vi "粘贴.vi"(8 "error in (no error)":errorcluster caption="错误输入（无错误）", 11 "程序 输入":refnum<class "程序.lvclass">) -> (0 "error out":errorcluster caption="错误输出", 3 "程序 输出":refnum<class "程序.lvclass">)   [LabVIEW 2020, in "程序.lvclass"]
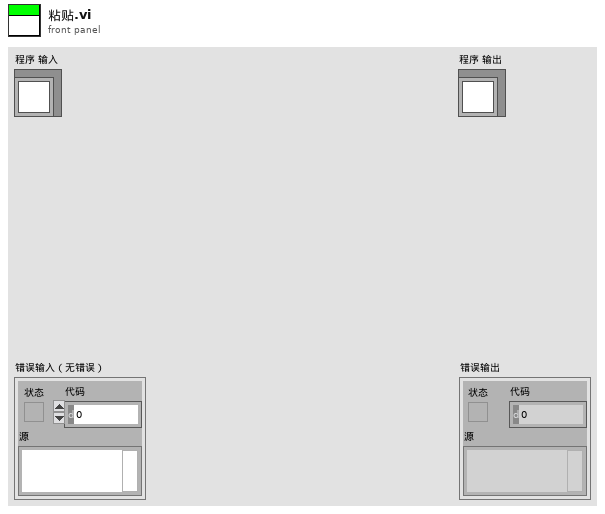
[diagram p1: front panel]
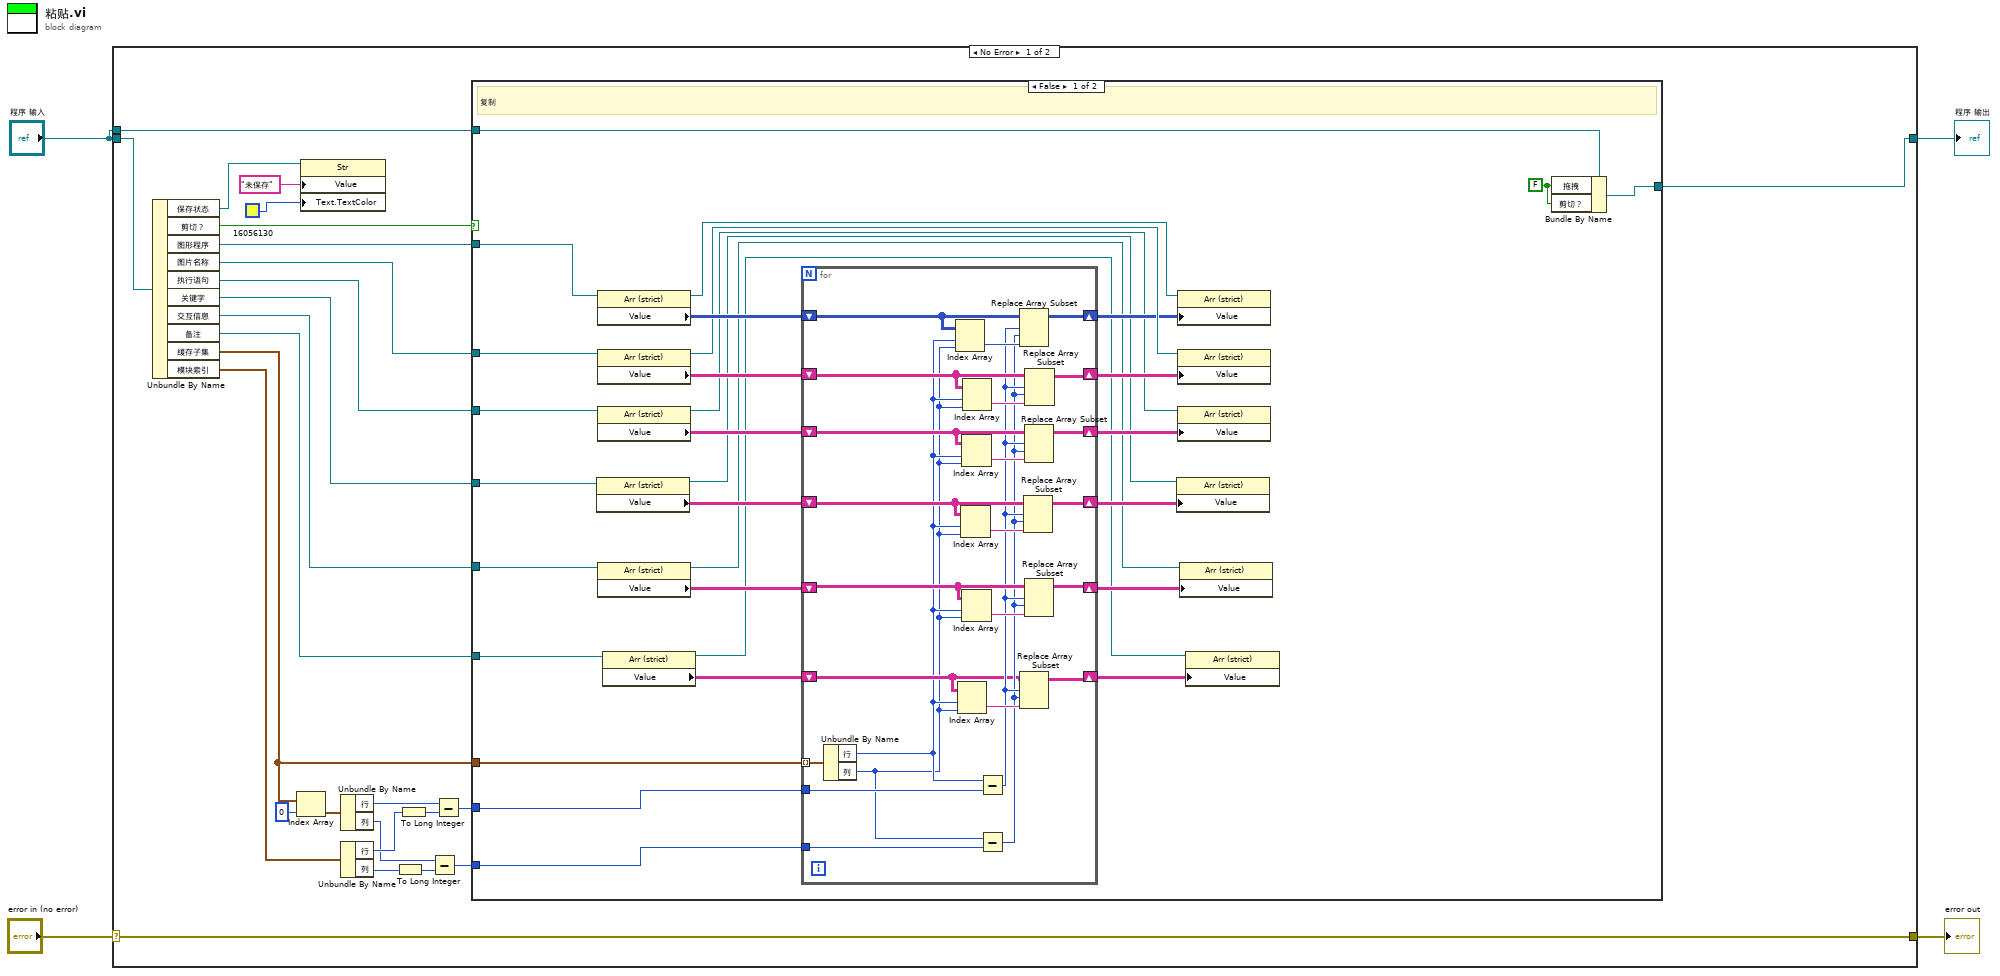
[diagram p0: block diagram]
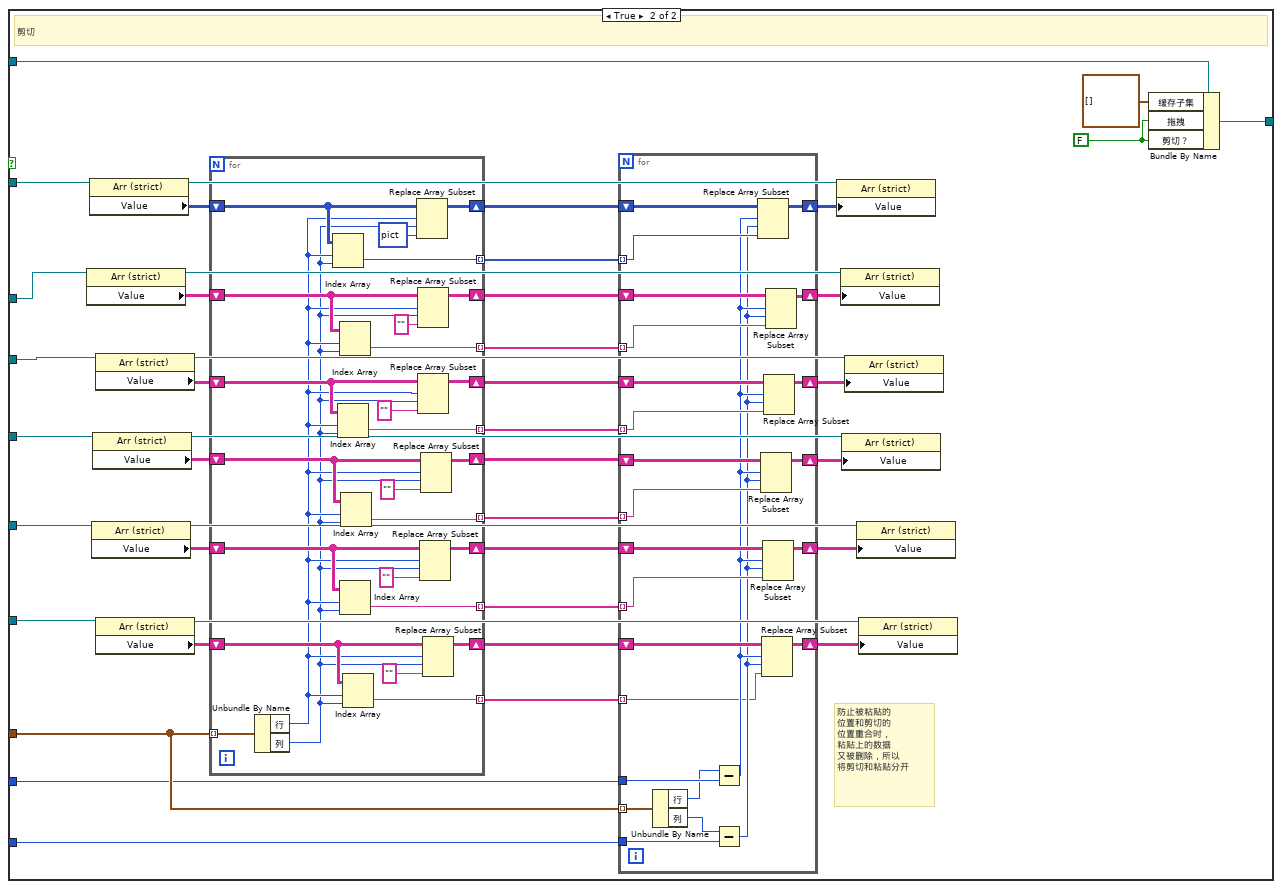
[diagram p2: hidden frame]
diagram:
  n1 = case shown="No Error" "error in (no error)" {
    selector: "error in (no error)" -> [w30 w182]
    tunnel: [w30 w182] -> w3
    tunnel: [w5 w181] -> w2
    tunnel: "程序 输入" -> [w7 w181]
    tunnel: "程序 输入" -> [w6 _]
    frame No Error {
      n2 = Unbundle By Name(w7) -> ("保存状态"=w8:refnum<vi>, "剪切？"=w19:bool, "图形程序"=w18:refnum<vi>, "图片名称"=w17:refnum<vi>, "执行语句"=w16:refnum<vi>, "关键字"=w13:refnum<vi>, "交互信息"=w12:refnum<vi>, "备注"=w11:refnum<vi>, "缓存子集"=w14:cluster{"行":i32, "列":i32}[], "模块索引"=w15:cluster{"列":u32, "行":u32})
      n3 = Index Array(array=w14, index=0 ("索引")) -> (element=w29:cluster{"行":i32, "列":i32})
      n4 = property class="Str"(reference=w8, "Value"="未保存" ("值"), "Text.TextColor"=u32 16056130) -> ()  [unwired: 1 in, 2 out]
      n5 = Unbundle By Name(w29) -> ("行"=w28:i32, "列"=w24:i32)
      n6 = Unbundle By Name(w15) -> ("行"=w27:u32, "列"=w23:u32)
      n7 = To Long Integer(number=w23) -> (32bit integer=w25:i32)
      n8 = To Long Integer(number=w27) -> (32bit integer=w26:i32)
      n9 = Subtract(x=w24, y=w25) -> (x-y=w21:i32)
      n10 = Subtract(x=w28, y=w26) -> (x-y=w22:i32)
      n11 = case shown="False" w19 {
        tunnel: w18 -> [w57 w121]
        tunnel: w17 -> [w55 w119]
        tunnel: w16 -> [w53 w116]
        tunnel: w14 -> [w58 w128]
        tunnel: w22 -> [w60 w124]
        tunnel: w21 -> [w59 w123]
        tunnel: w13 -> [w43 w106]
        tunnel: w12 -> [w41 w101]
        tunnel: w11 -> [w37 w95]
        tunnel: w6 -> [w33 w89]
        tunnel: [w32 w86] -> w5
        frame False {
          w31 = FALSE ("拖拽")
          # "复制"
          n12 = property class="Arr (strict)"(reference=w43) -> (reference out=w42:refnum<vi>, "Value"=w44:string[][])  [unwired: 1 in, 1 out]
          n13 = property class="Arr (strict)"(reference=w57) -> (reference out=w51:refnum<vi>, "Value"=w56:picture[][])  [unwired: 1 in, 1 out]
          n14 = property class="Arr (strict)"(reference=w55) -> (reference out=w48:refnum<vi>, "Value"=w54:string[][])  [unwired: 1 in, 1 out]
          n15 = property class="Arr (strict)"(reference=w53) -> (reference out=w46:refnum<vi>, "Value"=w52:string[][])  [unwired: 1 in, 1 out]
          n16 = property class="Arr (strict)"(reference=w41) -> (reference out=w39:refnum<vi>, "Value"=w40:string[][])  [unwired: 1 in, 1 out]
          n17 = property class="Arr (strict)"(reference=w37) -> (reference out=w34:refnum<vi>, "Value"=w36:string[][])  [unwired: 1 in, 1 out]
          n18 = for {
            tunnel: w58 -> [w85] mode=indexing
            tunnel: w60 -> [w84]
            tunnel: w59 -> [w83]
            shift-right: [w78] -> w47
            shift-left: w56 -> [w79]
            shift-right: [w76] -> w50
            shift-left: w54 -> [w77]
            shift-right: [w74] -> w49
            shift-left: w52 -> [w75]
            shift-right: [w73] -> w45
            shift-left: w44 -> [w72]
            shift-right: [w69] -> w38
            shift-left: w40 -> [w68]
            shift-right: [w66] -> w35
            shift-left: w36 -> [w63]
            n19 = Unbundle By Name(w85) -> ("行"=w62:i32, "列"=w61:i32)
            n20 = Index Array(array=w79, index (row)=w62, index (col)=w61) -> (element=w82:picture)
            n21 = Index Array(array=w63, index (row)=w62, index (col)=w61) -> (element=w67:string)
            n22 = Index Array(array=w72, index (row)=w62, index (col)=w61) -> (element=w71:string)
            n23 = Index Array(array=w75, index (row)=w62, index (col)=w61) -> (element=w80:string)
            n24 = Index Array(array=w68, index (row)=w62, index (col)=w61) -> (element=w70:string)
            n25 = Index Array(array=w77, index (row)=w62, index (col)=w61) -> (element=w81:string)
            n26 = Subtract(x=w62, y=w84) -> (x-y=w65:i32)
            n27 = Subtract(x=w61, y=w83) -> (x-y=w64:i32)
            n28 = Replace Array Subset(array=w79, new element=w82, index (row)=w65, index (col)=w64) -> (w78:picture[][])
            n29 = Replace Array Subset(array=w63, new element=w67, index (row)=w65, index (col)=w64) -> (w66:string[][])
            n30 = Replace Array Subset(array=w72, new element=w71, index (row)=w65, index (col)=w64) -> (w73:string[][])
            n31 = Replace Array Subset(array=w75, new element=w80, index (row)=w65, index (col)=w64) -> (w74:string[][])
            n32 = Replace Array Subset(array=w68, new element=w70, index (row)=w65, index (col)=w64) -> (w69:string[][])
            n33 = Replace Array Subset(array=w77, new element=w81, index (row)=w65, index (col)=w64) -> (w76:string[][])
          }
          n34 = property class="Arr (strict)"(reference=w42, "Value"=w45) -> ()  [unwired: 1 in, 2 out]
          n35 = property class="Arr (strict)"(reference=w51, "Value"=w47) -> ()  [unwired: 1 in, 2 out]
          n36 = property class="Arr (strict)"(reference=w48, "Value"=w50) -> ()  [unwired: 1 in, 2 out]
          n37 = property class="Arr (strict)"(reference=w46, "Value"=w49) -> ()  [unwired: 1 in, 2 out]
          n38 = property class="Arr (strict)"(reference=w39, "Value"=w38) -> ()  [unwired: 1 in, 2 out]
          n39 = property class="Arr (strict)"(reference=w34, "Value"=w35) -> ()  [unwired: 1 in, 2 out]
          n40 = Bundle By Name(cluster=w33, "拖拽"=w31, "剪切？"=w31) -> (w32:refnum<class "程序.lvclass">)
        }
        frame True {
          w87 = FALSE ("拖拽")
          # "防止被粘贴的\n位置和剪切的\n位置重合时，\n粘贴上的数据\n又被删除，所以\n将剪切和粘贴分开"
          # "剪切"
          n41 = property class="Arr (strict)"(reference=w119) -> (reference out=w109:refnum<vi>, "Value"=w118:string[][])  [unwired: 1 in, 1 out]
          n42 = property class="Arr (strict)"(reference=w121) -> (reference out=w110:refnum<vi>, "Value"=w120:picture[][])  [unwired: 1 in, 1 out]
          n43 = property class="Arr (strict)"(reference=w101) -> (reference out=w99:refnum<vi>, "Value"=w100:string[][])  [unwired: 1 in, 1 out]
          n44 = property class="Arr (strict)"(reference=w106) -> (reference out=w102:refnum<vi>, "Value"=w107:string[][])  [unwired: 1 in, 1 out]
          n45 = property class="Arr (strict)"(reference=w116) -> (reference out=w108:refnum<vi>, "Value"=w115:string[][])  [unwired: 1 in, 1 out]
          n46 = property class="Arr (strict)"(reference=w95) -> (reference out=w90:refnum<vi>, "Value"=w94:string[][])  [unwired: 1 in, 1 out]
          n47 = for {
            tunnel: w128 -> [w180] mode=indexing
            tunnel: [w177] -> w126 mode=indexing
            tunnel: [w176] -> w125 mode=indexing
            tunnel: [w175] -> w127 mode=indexing
            shift-right: [w174] -> w122
            shift-left: w120 -> [w173]
            shift-right: [w171] -> w117
            shift-left: w118 -> [w172]
            shift-right: [w169] -> w114
            shift-left: w115 -> [w170]
            tunnel: [w167] -> w103 mode=indexing
            shift-right: [w166] -> w104
            shift-left: w107 -> [w168]
            shift-right: [w162] -> w98
            shift-left: w100 -> [w161]
            tunnel: [w160] -> w97 mode=indexing
            shift-right: [w158] -> w92
            shift-left: w94 -> [w157]
            tunnel: [w154] -> w93 mode=indexing
            n48 = Unbundle By Name(w180) -> ("行"=w156:i32, "列"=w155:i32)
            n49 = Index Array(array=w173, index (row)=w156, index (col)=w155) -> (element=w176:picture)
            n50 = Index Array(array=w170, index (row)=w156, index (col)=w155) -> (element=w175:string)
            n51 = Index Array(array=w172, index (row)=w156, index (col)=w155) -> (element=w177:string)
            n52 = Index Array(array=w161, index (row)=w156, index (col)=w155) -> (element=w160:string)
            n53 = Index Array(array=w168, index (row)=w156, index (col)=w155) -> (element=w167:string)
            n54 = Index Array(array=w157, index (row)=w156, index (col)=w155) -> (element=w154:string)
            n55 = Replace Array Subset(array=w173, new element=picture data[5B] ("新元素/子数组"), index (row)=w156, index (col)=w155) -> (w174:picture[][])
            n56 = Replace Array Subset(array=w172, new element="" ("新元素/子数组"), index (row)=w156, index (col)=w155) -> (w171:string[][])
            n57 = Replace Array Subset(array=w170, new element="" ("新元素/子数组"), index (row)=w156, index (col)=w155) -> (w169:string[][])
            n58 = Replace Array Subset(array=w161, new element="" ("新元素/子数组"), index (row)=w156, index (col)=w155) -> (w162:string[][])
            n59 = Replace Array Subset(array=w168, new element="" ("新元素/子数组"), index (row)=w156, index (col)=w155) -> (w166:string[][])
            n60 = Replace Array Subset(array=w157, new element="" ("新元素/子数组"), index (row)=w156, index (col)=w155) -> (w158:string[][])
          }
          n61 = for {
            tunnel: w128 -> [w153] mode=indexing
            tunnel: w124 -> [w152]
            tunnel: w123 -> [w151]
            tunnel: w127 -> [w146] mode=indexing
            tunnel: w126 -> [w147] mode=indexing
            tunnel: w125 -> [w148] mode=indexing
            shift-right: [w144] -> w111
            shift-left: w122 -> [w145]
            shift-right: [w142] -> w112
            shift-left: w117 -> [w143]
            shift-right: [w140] -> w113
            shift-left: w114 -> [w141]
            tunnel: w103 -> [w137] mode=indexing
            shift-right: [w139] -> w105
            shift-left: w104 -> [w138]
            tunnel: w97 -> [w134] mode=indexing
            shift-right: [w135] -> w96
            shift-left: w98 -> [w136]
            tunnel: w93 -> [w129] mode=indexing
            shift-right: [w132] -> w91
            shift-left: w92 -> [w133]
            n62 = Unbundle By Name(w153) -> ("行"=w150:i32, "列"=w149:i32)
            n63 = Subtract(x=w150, y=w152) -> (x-y=w131:i32)
            n64 = Subtract(x=w149, y=w151) -> (x-y=w130:i32)
            n65 = Replace Array Subset(array=w145, new element=w148, index (row)=w131, index (col)=w130) -> (w144:picture[][])
            n66 = Replace Array Subset(array=w138, new element=w137, index (row)=w131, index (col)=w130) -> (w139:string[][])
            n67 = Replace Array Subset(array=w133, new element=w129, index (row)=w131, index (col)=w130) -> (w132:string[][])
            n68 = Replace Array Subset(array=w136, new element=w134, index (row)=w131, index (col)=w130) -> (w135:string[][])
            n69 = Replace Array Subset(array=w141, new element=w146, index (row)=w131, index (col)=w130) -> (w140:string[][])
            n70 = Replace Array Subset(array=w143, new element=w147, index (row)=w131, index (col)=w130) -> (w142:string[][])
          }
          n71 = property class="Arr (strict)"(reference=w110, "Value"=w111) -> ()  [unwired: 1 in, 2 out]
          n72 = property class="Arr (strict)"(reference=w109, "Value"=w112) -> ()  [unwired: 1 in, 2 out]
          n73 = property class="Arr (strict)"(reference=w102, "Value"=w105) -> ()  [unwired: 1 in, 2 out]
          n74 = property class="Arr (strict)"(reference=w108, "Value"=w113) -> ()  [unwired: 1 in, 2 out]
          n75 = property class="Arr (strict)"(reference=w99, "Value"=w96) -> ()  [unwired: 1 in, 2 out]
          n76 = property class="Arr (strict)"(reference=w90, "Value"=w91) -> ()  [unwired: 1 in, 2 out]
          n77 = Bundle By Name(cluster=w89, "缓存子集"=cluster{"行":i32, "列":i32}[] [], "拖拽"=w87, "剪切？"=w87) -> (w86:refnum<class "程序.lvclass">)
        }
      }
    }
    frame Error {
    }
  }
  "error out" <- w3
  "程序 输出" <- w2
